vi "AddTestMethod_Provider_Interface.vi"() -> (3 "Interface Table":T1)   [LabVIEW 2013]
uses:
  <resource>/Framework/Providers/API/Provider_Interface.ctl
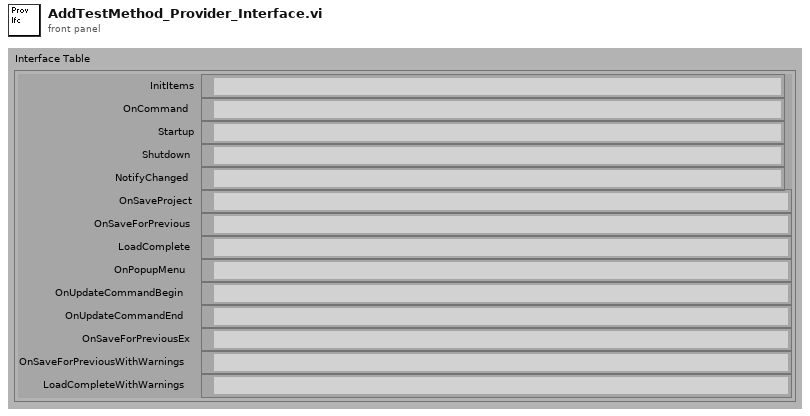
[diagram p1: front panel]
types:
  T1 = typedef "Provider_Interface.ctl" = cluster{"InitItems":path, "OnCommand":path, "Startup":path, "Shutdown":path, "NotifyChanged":path, "OnSaveProject":path, "OnSaveForPrevious":path, "LoadComplete":path, "OnPopupMenu":path, "OnUpdateCommandBegin":path, "OnUpdateCommandEnd":path, "OnSaveForPreviousEx":path, "OnSaveForPreviousWithWarnings":path, "LoadCompleteWithWarnings":path}
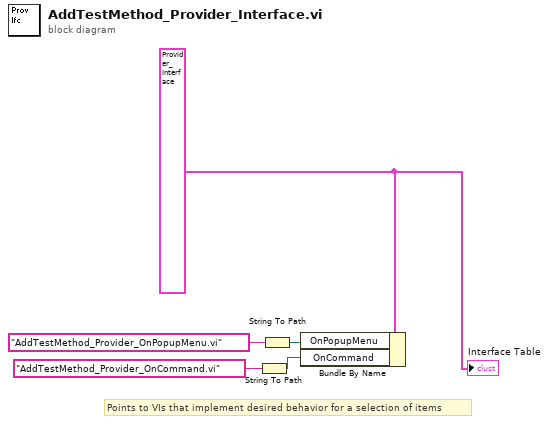
[diagram p0: block diagram]
diagram:
  w1 = T1 {"InitItems"=path "", "OnCommand"=path "", "Startup"=path "", "Shutdown"=path "", "NotifyChanged"=path "", "OnSaveProject"=path "", "OnSaveForPrevious"=path "", "LoadComplete"=path "", "OnPopupMenu"=path "", "OnUpdateCommandBegin"=path "", "OnUpdateCommandEnd"=path "", "OnSaveForPreviousEx"=path "", "OnSaveForPreviousWithWarnings"=path "", "LoadCompleteWithWarnings"=path ""} ("InterfaceTable")
  # "Points to VIs that implement desired behavior for a selection of items"
  n1 = String To Path(string="AddTestMethod_Provider_OnCommand.vi") -> (path=w3:path)
  n2 = String To Path(string="AddTestMethod_Provider_OnPopupMenu.vi") -> (path=w5:path)
  n3 = Bundle By Name(cluster=w1, "OnPopupMenu"=w5, "OnCommand"=w3) -> ()  [unwired: 1 out]
  "Interface Table" <- w1
